vi "3PhaseSPWM.vi"() -> ()   [LabVIEW 2016]
uses:
  <vilib>/Instr/_visa.llb/VISA Configure Serial Port (Instr).vi
panel:
  in  "Maple Motor Controller":enum32{"MOTOR CONTROLLER", "SETTINGS"}(tab)
  out "Boolean 2":bool
  in  "UPDATE":bool
  in  "PWM FREQUENCY":sgl[unit](knob)=100.0 min=1 max=3500 step=1 scale=1.0..3500.0 scale format="%#_6f"
  in  "CENTER \nALIGNED":bool=TRUE
  out "Boolean 4":bool=TRUE
  in  "CH4":u16(knob)=10 max=100 scale=0.0..100.0
  in  "CH3":u16(knob)=30 max=100 scale=0.0..100.0
  in  "CH2":u16(knob)=50 max=100 scale=0.0..100.0
  in  "CH1":u16(knob)=80 max=100 scale=0.0..100.0
  in  "SPWM FREQUENCY":dbl[unit](knob)=44.0 min=1.0 max=1000.0 scale=1.0..1000.0 scale format="%#_6f"
  in  "3-PHASE SPWM":bool
  out "Boolean 3":bool
  out "VISA resource name out":refnum<visa-resource-name>="COM3"
  out "comp_val_ch1":u16=562
  out "arr_val":u16=702
  in  "timeout (10sec)":u32=10000
  out "serial_out_string":string="702;1024;562;351;211;70;1349097;1;0;#"
  out "pre_scaler":u16=1024
  out "tuning_word":dbl=1349096.9592759225
  in  "VISA resource name":refnum<visa-resource-name>="COM3"
  out "comp_val_ch2":u16=351
  out "comp_val_ch3":u16=211
  out "comp_val_ch4":u16=70
  # "DUTY CYCLE"
  # "%"
  # "%"
  # "%"
  # "%"
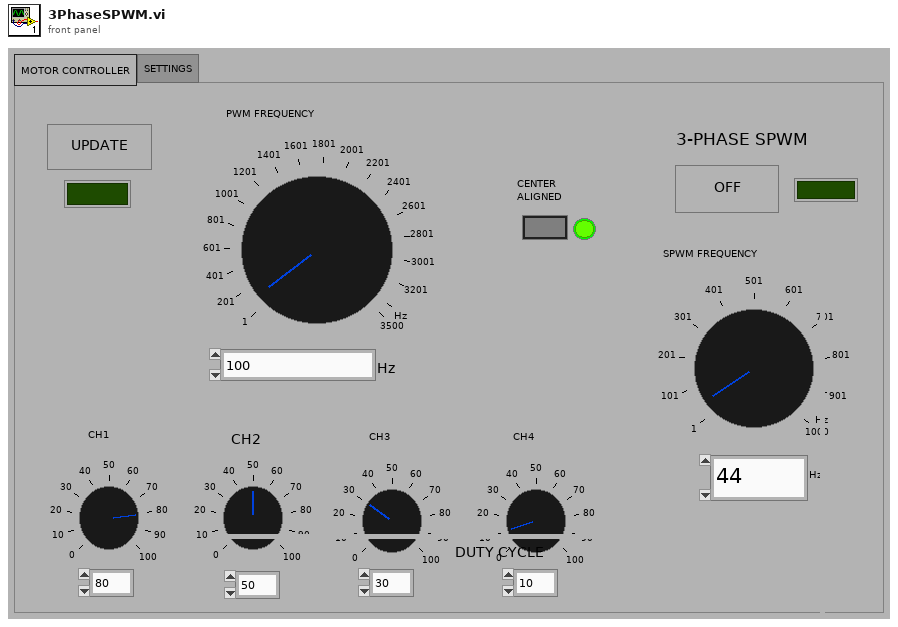
[diagram p1: front panel]
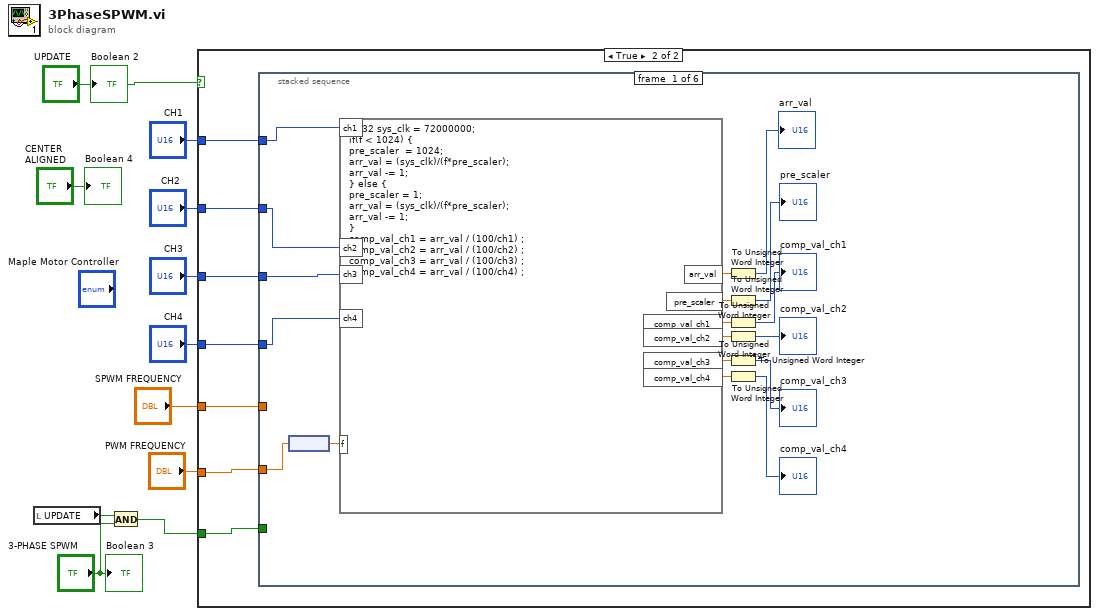
[diagram p0: block diagram]
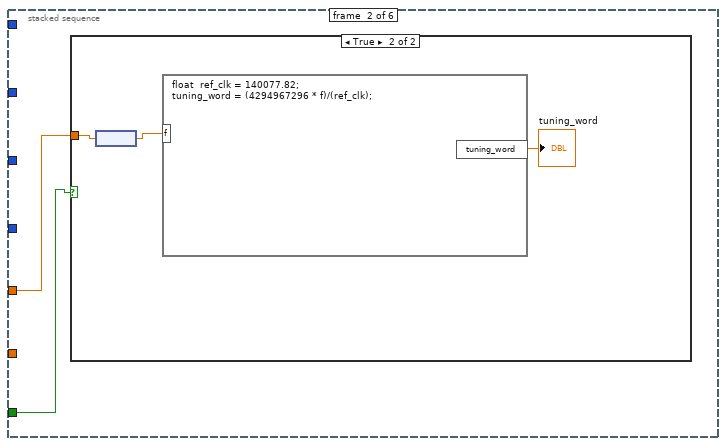
[diagram p3: hidden frame]
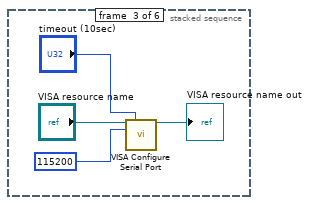
[diagram p5: hidden frame]
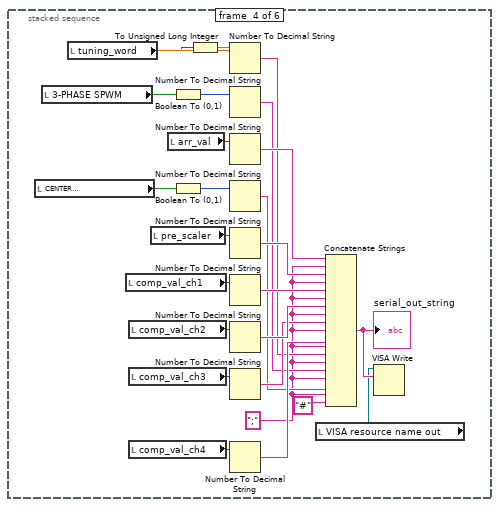
[diagram p6: hidden frame]
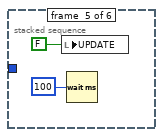
[diagram p7: hidden frame]
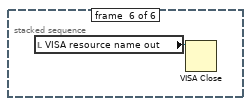
[diagram p8: hidden frame]
diagram:
  n1 = local read "UPDATE"() -> (w5:bool)
  n2 = And(x=w5, y="3-PHASE SPWM") -> (x .and. y?=w2:bool)
  n3 = case shown="True" "UPDATE" {
    tunnel: "PWM FREQUENCY" -> [_ w14]
    tunnel: "CH1" -> [_ w18]
    tunnel: "CH3" -> [_ w17]
    tunnel: "CH2" -> [_ w16]
    tunnel: "CH4" -> [_ w15]
    tunnel: w2 -> [_ w13]
    tunnel: "SPWM FREQUENCY" -> [_ w12]
    frame False {
    }
    frame True {
      n4 = stacked-sequence {
        tunnel: w18 -> [w30 _ _ _ _ _]
        tunnel: w17 -> [w28 _ _ _ _ _]
        tunnel: w16 -> [w29 _ _ _ _ _]
        tunnel: w15 -> [w27 _ _ _ _ _]
        tunnel: w14 -> [w20 _ _ _ _ _]
        tunnel: w13 -> [_ w38 _ _ _ _]
        tunnel: w12 -> [_ w37 _ _ _ _]
        frame #0 {
          n5 = node(w20) -> (w19:sgl)
          n6 = formula code="int32 sys_clk = 72000000;\nif(f < 1024) {\npre_scaler  = 1024;\narr_val = (sys_clk)/(f*pre_scaler);\narr_val -= 1;\n} else {\npre_scaler = 1;\narr_val = (sys_clk)/(f*pre_scaler);\narr_val -= 1;\n}\ncomp_val_ch1 = arr_val / (100/ch1) ;\ncomp_val_ch2 = arr_val / (100/ch2) ;\ncomp_val_ch3 = arr_val / (100/ch3) ;\ncomp_val_ch4 = arr_val / (100/ch4) ;"("ch1"=w30, "f"=w19, "ch2"=w29, "ch3"=w28, "ch4"=w27) -> ("arr_val"=w34:dbl, "pre_scaler"=w36:dbl, "comp_val_ch1"=w35:dbl, "comp_val_ch2"=w26:dbl, "comp_val_ch3"=w25:dbl, "comp_val_ch4"=w24:dbl)
          n7 = To Unsigned Word Integer(number=w34) -> (unsigned 16bit integer=→"arr_val":u16)
          n8 = To Unsigned Word Integer(number=w36) -> (unsigned 16bit integer=→"pre_scaler":u16)
          n9 = To Unsigned Word Integer(number=w35) -> (unsigned 16bit integer=→"comp_val_ch1":u16)
          n10 = To Unsigned Word Integer(number=w26) -> (unsigned 16bit integer=→"comp_val_ch2":u16)
          n11 = To Unsigned Word Integer(number=w25) -> (unsigned 16bit integer=→"comp_val_ch3":u16)
          n12 = To Unsigned Word Integer(number=w24) -> (unsigned 16bit integer=→"comp_val_ch4":u16)
        }
        frame #1 {
          n13 = case shown="True" w38 {
            tunnel: w37 -> [_ w40]
            frame False {
            }
            frame True {
              n14 = node(w40) -> (w39:dbl)
              n15 = formula code="float  ref_clk = 140077.82;\ntuning_word = (4294967296 * f)/(ref_clk);"("f"=w39) -> ("tuning_word"=→"tuning_word":dbl)
            }
          }
        }
        frame #2 {
          n16 = call-poly "VISA Configure Serial Port"("VISA resource name"="VISA resource name", "timeout (10sec)"="timeout (10sec)", "baud rate (9600)"=u32 115200) -> ("VISA resource name out"=→"VISA resource name out":refnum<visa-resource-name>)  [unwired: 4 in, 8 out]
        }
        frame #3 {
          w47 = ";" ("string")
          n17 = local read "CENTER \nALIGNED"() -> (w51:bool)
          n18 = local read "3-PHASE SPWM"() -> (w66:bool)
          n19 = local read "tuning_word"() -> (w64:dbl)
          n20 = local read "comp_val_ch1"() -> (w67:u16)
          n21 = local read "comp_val_ch2"() -> (w60:u16)
          n22 = local read "comp_val_ch3"() -> (w59:u16)
          n23 = local read "comp_val_ch4"() -> (w58:u16)
          n24 = local read "pre_scaler"() -> (w68:u16)
          n25 = local read "arr_val"() -> (w69:u16)
          n26 = Boolean To (0,1)(Boolean=w66) -> (0, 1=w65:i16)
          n27 = Boolean To (0,1)(Boolean=w51) -> (0, 1=w50:i16)
          n28 = To Unsigned Long Integer(number=w64) -> (unsigned 32bit integer=w63:u32)
          n29 = Number To Decimal String(number=w63) -> (decimal integer string=w52:string)  [unwired: 1 out]
          n30 = Number To Decimal String(number=w65) -> (decimal integer string=w49:string)  [unwired: 1 out]
          n31 = Number To Decimal String(number=w69) -> (decimal integer string=w61:string)  [unwired: 1 out]
          n32 = Number To Decimal String(number=w50) -> (decimal integer string=w48:string)  [unwired: 1 out]
          n33 = Number To Decimal String(number=w68) -> (decimal integer string=w57:string)  [unwired: 1 out]
          n34 = Number To Decimal String(number=w67) -> (decimal integer string=w56:string)  [unwired: 1 out]
          n35 = Number To Decimal String(number=w60) -> (decimal integer string=w55:string)  [unwired: 1 out]
          n36 = Number To Decimal String(number=w59) -> (decimal integer string=w54:string)  [unwired: 1 out]
          n37 = Number To Decimal String(number=w58) -> (decimal integer string=w53:string)  [unwired: 1 out]
          n38 = local read "VISA resource name out"() -> (w62:refnum<visa-resource-name>)
          n39 = Concatenate Strings(w61, w47, w57, w47, w56, w47, w55, w47, w54, w47, w53, w47, w52, w47, w49, w47, w48, w47, "#" ("string")) -> (w70:string)
          "serial_out_string" <- w70
          n40 = VISA Write(VISA resource name=w62, write buffer=w70) -> ()  [unwired: 1 in, 3 out]
        }
        frame #4 {
          n41 = local write "UPDATE"(FALSE ("Boolean")) -> ()
          n42 = Wait (ms)(milliseconds to wait=u32 100) -> ()  [unwired: 1 out]
        }
        frame #5 {
          n43 = local read "VISA resource name out"() -> (w73:refnum<visa-resource-name>)
          n44 = VISA Close(VISA resource name=w73) -> ()  [unwired: 1 in, 1 out]
        }
      }
    }
  }
  "Boolean 2" <- "UPDATE"
  "Boolean 3" <- "3-PHASE SPWM"
  "Boolean 4" <- "CENTER \nALIGNED"
